vi "instr.RelayBD_V03_PT_SCPI.vi"(6 "测试日志信息":refnum<queue>, 7 "timeout (10sec)":u32=1000 caption="超时（10秒）", 8 "error in (no error)":errorcluster caption="错误输入（无错误）", 9 "CMD_SCPI":string, 10 "baud rate (9600)":u32=9600 caption="波特率(9600)", 11 "VISA resource name":refnum<visa-resource-name>="COM1" caption="VISA资源名称") -> (0 "error out":errorcluster caption="错误输出", 2 "返回字符串":string, 3 "OK?":bool, 4 "发送字符串":string)   [LabVIEW 2012, in "Lib_UEL.ATE.lvlib" / "Lib_Instrument.lvlib"]
uses:
  Lib_Instrument.lvlib
  <vilib>/Instr/_visa.llb/VISA Configure Serial Port (Instr).vi
panel:
  # "支持的SCPI命令:\nCONTROL_SET_ALL\nCONTROL_SET_RELAYA1 \nCONTROL_SET_RELAYA8 \nCONTROL_SET_RELAYB1 \nCONTROL_SET_RELAYB8 \nMEASURE_READ_CHANA  \nMEASURE_READ_CHAND  \nSYSCMD_IDN          \nSYSCMD_RST          \nSYSTEM_VERSION"
  # "2014-7-11,V01\n- HW:RelayBDV03,SW:PT1.4+SCPI"
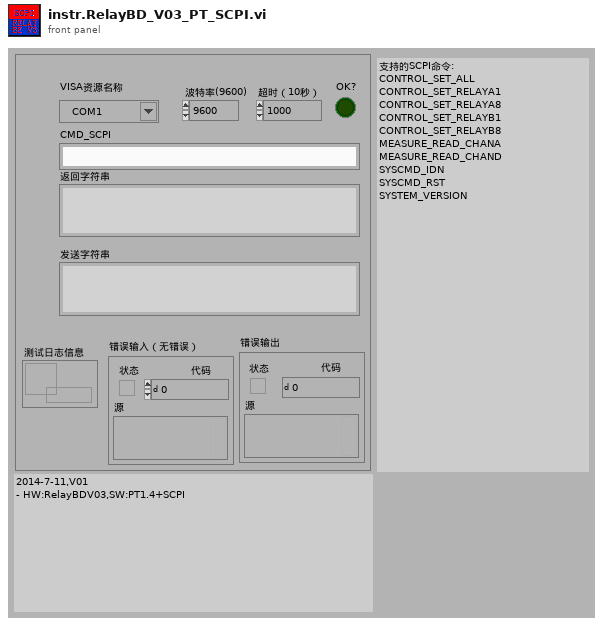
[diagram p1: front panel]
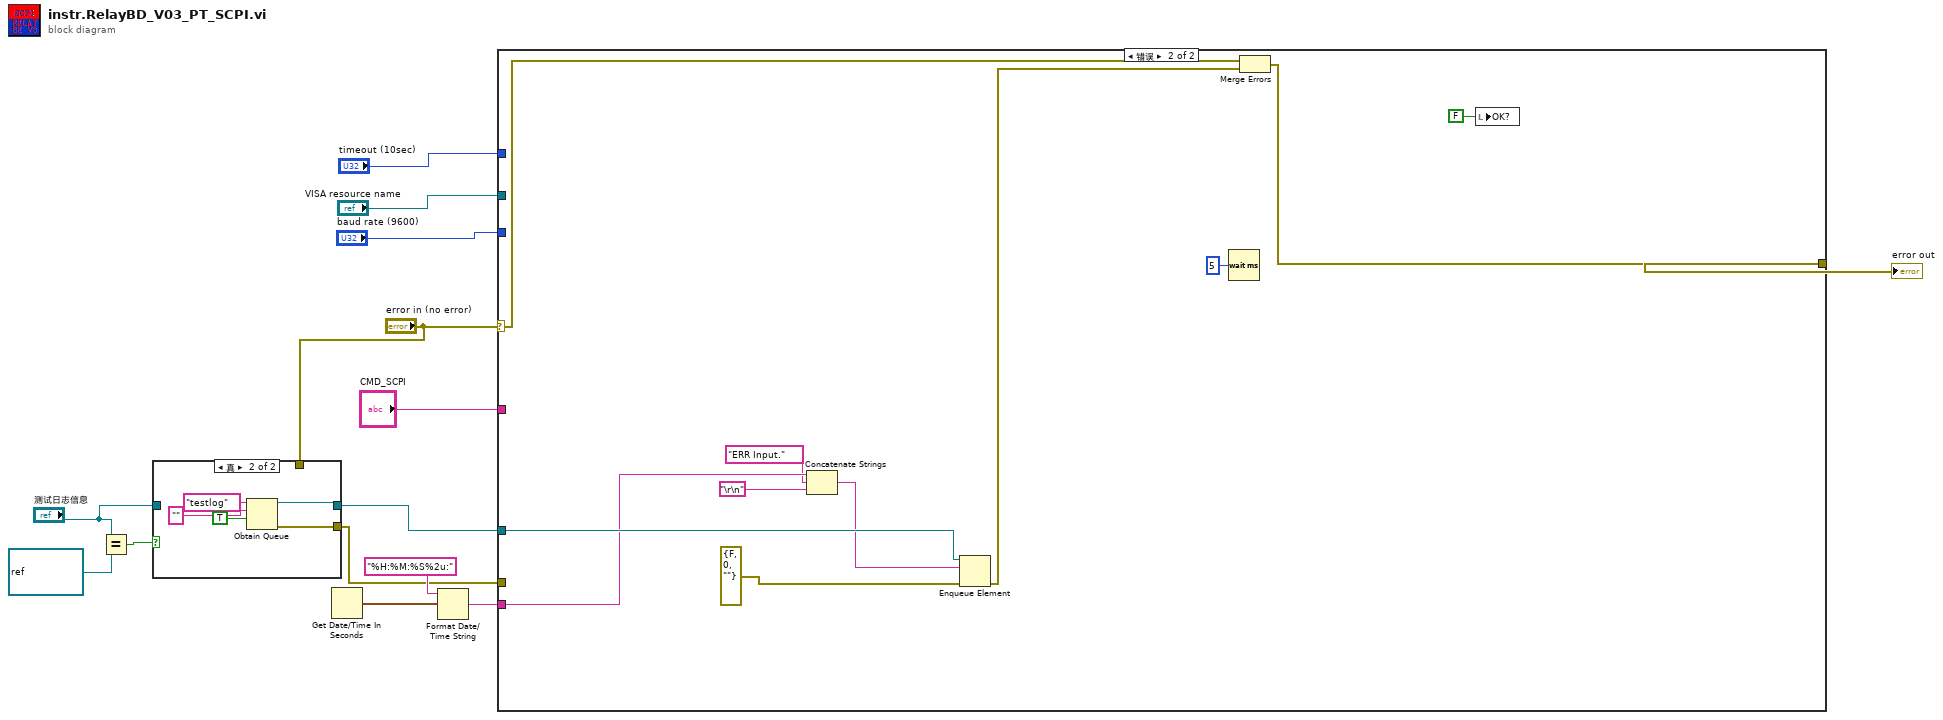
[diagram p0: block diagram]
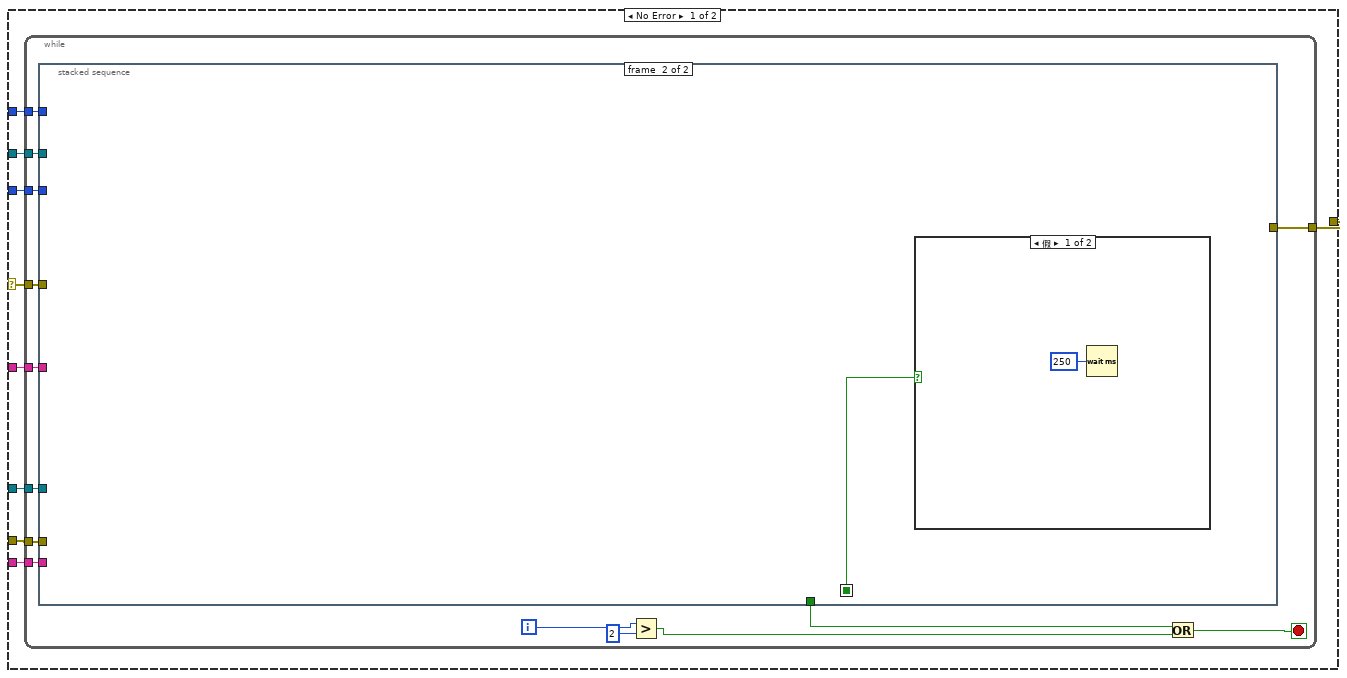
[diagram p3: hidden frame]
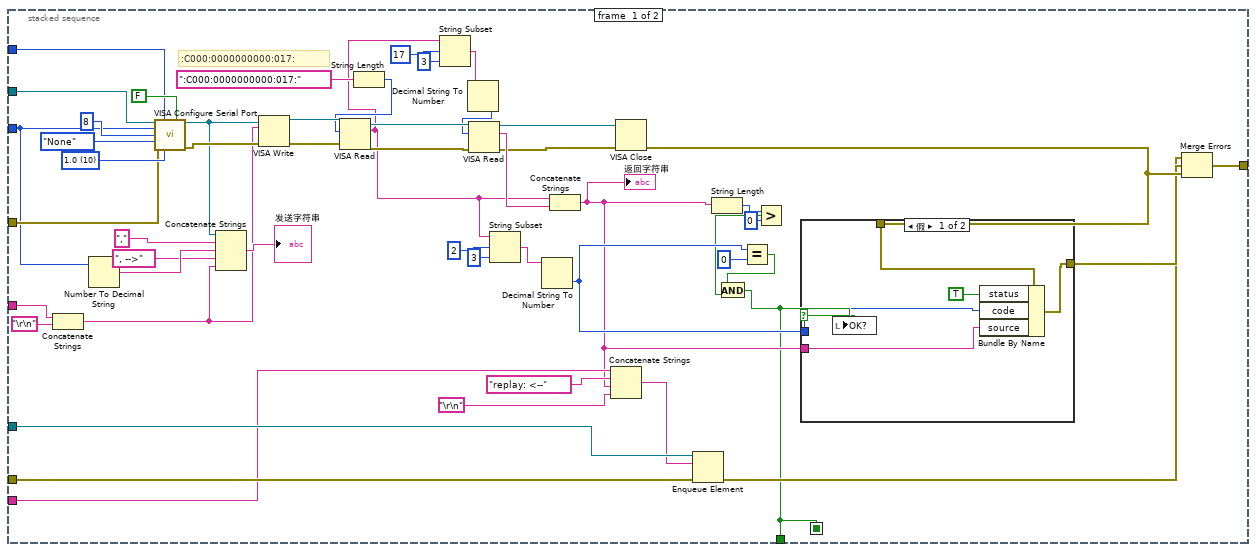
[diagram p4: hidden frame]
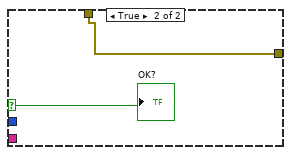
[diagram p5: hidden frame]
diagram:
  n1 = Equal?(x="测试日志信息", y=refnum<queue> refnum) -> (x = y?=w6:bool)
  n2 = case shown="真" w6 {
    tunnel: "测试日志信息" -> [w16 _]
    tunnel: [w16 w21] -> w4
    tunnel: [w15 w20] -> w2
    tunnel: "error in (no error)" -> [w15 _]
    frame False {
    }
    frame True {
      n3 = Obtain Queue(name (unnamed)="testlog" ("名称（未命名）"), element data type="" ("名称（未命名）"), create if not found? (T)=TRUE ("如未找到是否创建？(T)")) -> (queue out=w21:refnum<queue>, error out=w20:errorcluster)  [unwired: 2 in, 1 out]
    }
  }
  n4 = Get Date/Time In Seconds() -> (seconds since 1Jan1904=w9:timestamp)
  n5 = Format Date/Time String(time format string (%c)="%H:%M:%S%2u:" ("时间格式化字符串(%c)"), seconds (now)=w9) -> (date/time string=w8:string)  [unwired: 1 in]
  n6 = case shown="错误" "error in (no error)" {
    selector: "error in (no error)" -> [w28 w114]
    tunnel: "VISA resource name" -> [w30 _]
    tunnel: [w27 w113] -> w11
    tunnel: "baud rate (9600)" -> [w26 _]
    tunnel: "timeout (10sec)" -> [w29 _]
    tunnel: w2 -> [w24 _]
    tunnel: w4 -> [w25 w112]
    tunnel: w8 -> [w23 w111]
    tunnel: "CMD_SCPI" -> [w22 _]
    frame No Error {
      n7 = while {
        tunnel: w30 -> [w44]
        tunnel: w29 -> [w43]
        tunnel: w28 -> [w42]
        tunnel: [w41] -> w27
        tunnel: w26 -> [w40]
        tunnel: w25 -> [w39]
        tunnel: w24 -> [w38]
        tunnel: w23 -> [w37]
        tunnel: w22 -> [w36]
        i -> [w33]
        stop <- w35 stop-if-true
        n8 = stacked-sequence {
          seq-local: [w45 _] -> [_ w105]
          tunnel: w44 -> [w96 _]
          tunnel: w43 -> [w91 _]
          tunnel: w42 -> [w88 _]
          tunnel: [w82 _] -> w41
          tunnel: w40 -> [w81 _]
          tunnel: w39 -> [w77 _]
          tunnel: w38 -> [w76 _]
          tunnel: w37 -> [w75 _]
          tunnel: w36 -> [w50 _]
          tunnel: [w45 _] -> w34
          frame #0 {
            w89 = u16 10 items=["1.0"=10, "1.5"=15, "2.0"=20] ("stop bits (10: 1 bit)")
            # ":C000:0000000000:017:"
            n9 = Concatenate Strings(w50, "\r\n") -> (w48:string)
            n10 = Number To Decimal String(number=w81) -> (decimal integer string=w79:string)  [unwired: 1 in]
            n11 = call-poly "VISA Configure Serial Port"("VISA resource name"=w96, "timeout (10sec)"=w91, "Enable Termination\nChar (T)"=FALSE ("Enable Termination\nChar (T)"), "baud rate (9600)"=w81, "data bits (8)"=u16 8, "parity (0:none)"=enum16{"None", "Odd", "Even", "Mark", "Space"}."None", "error in (no error)"=w88, "stop bits (10: 1 bit)"=w89) -> ("VISA resource name out"=w80:refnum<visa-resource-name>, "error out"=w87:errorcluster)  [unwired: 6 in]
            n12 = Concatenate Strings(w80, "," ("字符串"), w79, ", -->" ("字符串"), w48) -> (→"发送字符串":string)
            n13 = VISA Write(VISA resource name=w80, write buffer=w48, error in (no error)=w87) -> (VISA resource name out=w94:refnum<visa-resource-name>, error out=w93:errorcluster)  [unwired: 1 out]
            n14 = String Length(string=":C000:0000000000:017:" ("字符串")) -> (length=w69:i32)
            n15 = VISA Read(VISA resource name=w94, byte count=w69, error in (no error)=w93) -> (VISA resource name out=w85:refnum<visa-resource-name>, read buffer=w46:string, error out=w86:errorcluster)  [unwired: 1 out]
            n16 = String Subset(string=w46, offset (0)=17 ("偏移量(0)"), length (rest)=3 ("长度（剩余）")) -> (substring=w47:string)
            n17 = Decimal String To Number(string=w47) -> (number=w66:i32)  [unwired: 2 in, 1 out]
            n18 = VISA Read(VISA resource name=w85, byte count=w66, error in (no error)=w86) -> (VISA resource name out=w63:refnum<visa-resource-name>, read buffer=w65:string, error out=w64:errorcluster)  [unwired: 1 out]
            n19 = String Subset(string=w46, offset (0)=2 ("偏移量(0)"), length (rest)=3 ("长度（剩余）")) -> (substring=w58:string)
            n20 = Decimal String To Number(string=w58) -> (number=w56:i32)  [unwired: 2 in, 1 out]
            n21 = Concatenate Strings(w46, w65) -> (w55:string)
            "返回字符串" <- w55
            n22 = Concatenate Strings(w75, "replay: <--" ("字符串"), w55, "\r\n") -> (w74:string)
            n23 = VISA Close(VISA resource name=w63, error in (no error)=w64) -> (error out=w84:errorcluster)
            n24 = Enqueue Element(queue=w77, element=w74, error in (no error)=w76) -> (error out=w73:errorcluster)  [unwired: 1 in, 2 out]
            n25 = String Length(string=w55) -> (length=w54:i32)
            n26 = Equal?(x=w56, y=0) -> (x = y?=w51:bool)
            n27 = Greater?(x=w54, y=0) -> (0:w52:bool)
            n28 = And(x=w51, y=w52) -> (x .and. y?=w45:bool)
            n29 = case shown="假" w45 {
              selector: w45 -> [w102 w104]
              tunnel: [w99 w103] -> w83
              tunnel: w84 -> [w101 w103]
              tunnel: w56 -> [w98 _]
              tunnel: w55 -> [w97 _]
              frame False {
                n30 = local write "OK?"(w102) -> ()
                n31 = Bundle By Name(cluster=w101, "status"=TRUE, "code"=w98, "source"=w97) -> (w99:errorcluster)
              }
              frame True {
                "OK?" <- w104
              }
            }
            n32 = Merge Errors(w73, w83, w84) -> (w82:errorcluster)
          }
          frame #1 {
            n33 = case shown="假" w105 {
              frame False {
                n34 = Wait (ms)(milliseconds to wait=u32 250 ("等待时间（毫秒）")) -> ()  [unwired: 1 out]
              }
              frame True {
              }
            }
          }
        }
        n35 = Greater?(x=w33, y=2) -> (0:w31:bool)
        n36 = Or(x=w34, y=w31) -> (x .or. y?=w35:bool)
      }
    }
    frame Error {
      n37 = Concatenate Strings(w111, "ERR Input." ("字符串"), "\r\n") -> (w108:string)
      n38 = Enqueue Element(queue=w112, element=w108, error in (no error)=errorcluster {"status"=FALSE, "code"=0, "source"=""} ("错误输入（无错误）")) -> (error out=w115:errorcluster)  [unwired: 1 in, 2 out]
      n39 = Wait (ms)(milliseconds to wait=u32 5 ("等待时间（毫秒）")) -> ()  [unwired: 1 out]
      n40 = Merge Errors(w114, w115) -> (w113:errorcluster)
      n41 = local write "OK?"(FALSE ("OK?")) -> ()
    }
  }
  "error out" <- w11
